vi "TimedCaseIndex.vi"(10 "CaseTimes":u32[](array[numeric]), 11 "ElapsedTime":u32) -> (3 "CaseNumber":u32)   [LabVIEW 2017]
panel:
  out "Numeric":i32
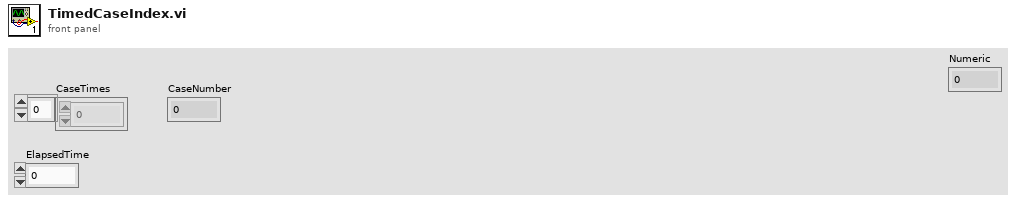
[diagram p1: front panel]
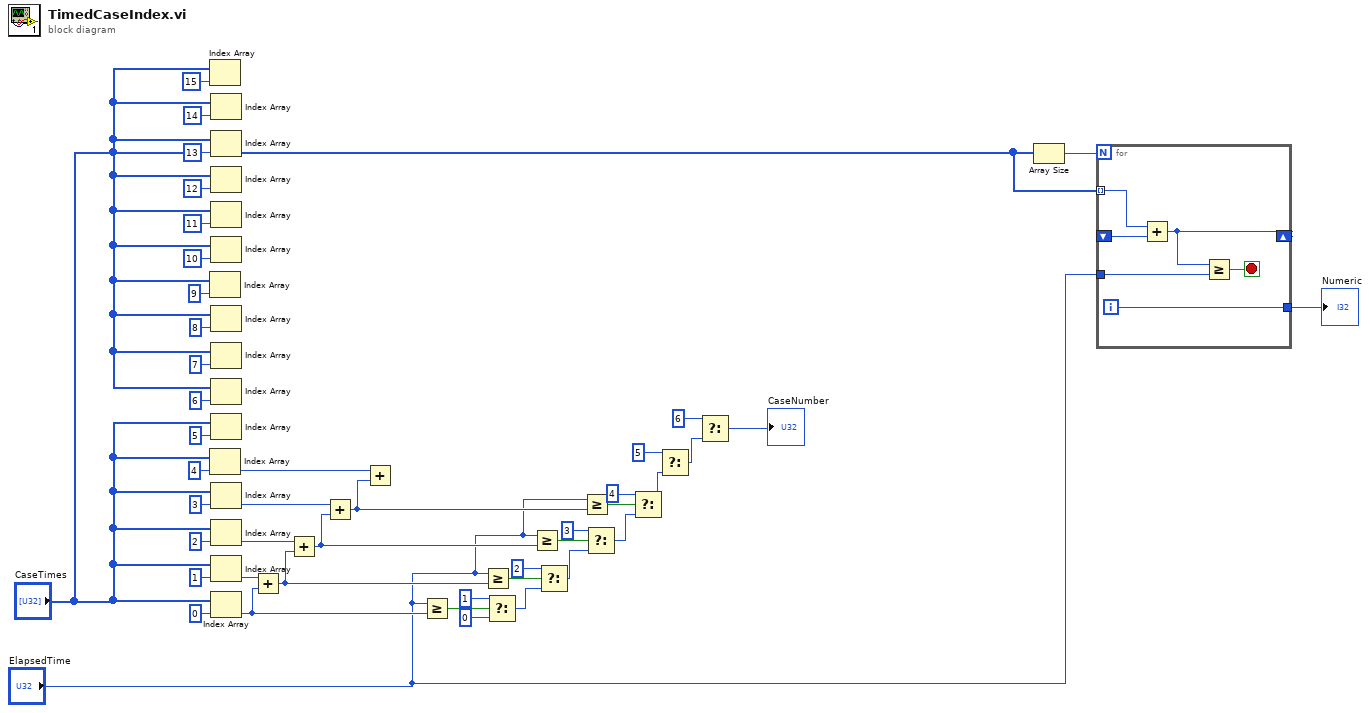
[diagram p0: block diagram]
diagram:
  n1 = Index Array(array="CaseTimes", index=15) -> ()  [unwired: 1 out]
  n2 = Index Array(array="CaseTimes", index=9) -> ()  [unwired: 1 out]
  n3 = Index Array(array="CaseTimes", index=4) -> (element=w6:u32)
  n4 = Index Array(array="CaseTimes", index=14) -> ()  [unwired: 1 out]
  n5 = Index Array(array="CaseTimes", index=13) -> ()  [unwired: 1 out]
  n6 = Index Array(array="CaseTimes", index=12) -> ()  [unwired: 1 out]
  n7 = Index Array(array="CaseTimes", index=11) -> ()  [unwired: 1 out]
  n8 = Index Array(array="CaseTimes", index=10) -> ()  [unwired: 1 out]
  n9 = Index Array(array="CaseTimes", index=8) -> ()  [unwired: 1 out]
  n10 = Index Array(array="CaseTimes", index=7) -> ()  [unwired: 1 out]
  n11 = Index Array(array="CaseTimes", index=6) -> ()  [unwired: 1 out]
  n12 = Index Array(array="CaseTimes", index=5) -> ()  [unwired: 1 out]
  n13 = Index Array(array="CaseTimes", index=3) -> (element=w10:u32)
  n14 = Index Array(array="CaseTimes", index=2) -> (element=w12:u32)
  n15 = Index Array(array="CaseTimes", index=1) -> (element=w15:u32)
  n16 = Index Array(array="CaseTimes", index=0) -> (element=w16:u32)
  n17 = Add(x=w15, y=w16) -> (x+y=w11:u32)
  n18 = Add(x=w12, y=w11) -> (x+y=w9:u32)
  n19 = Add(x=w10, y=w9) -> (x+y=w5:u32)
  n20 = Add(x=w6, y=w5) -> ()  [unwired: 1 out]
  n21 = Greater Or Equal?(x="ElapsedTime", y=w16) -> (x >= y?=w14:bool)
  n22 = Greater Or Equal?(x="ElapsedTime", y=w11) -> (x >= y?=w13:bool)
  n23 = Select(t=u32 1, s=w14, f=u32 0) -> (s? t:f=w41:u32)
  n24 = Greater Or Equal?(x="ElapsedTime", y=w9) -> (x >= y?=w8:bool)
  n25 = Select(t=u32 2, s=w13, f=w41) -> (s? t:f=w31:u32)
  n26 = Greater Or Equal?(x="ElapsedTime", y=w5) -> (x >= y?=w7:bool)
  n27 = Select(t=u32 3, s=w8, f=w31) -> (s? t:f=w32:u32)
  n28 = Select(t=u32 4, s=w7, f=w32) -> (s? t:f=w33:u32)
  n29 = Select(t=u32 5, f=w33) -> (s? t:f=w27:u32)  [unwired: 1 in]
  n30 = Select(t=u32 6, f=w27) -> (s? t:f=→"CaseNumber":u32)  [unwired: 1 in]
  n31 = Array Size(array="CaseTimes") -> (size(s)=w4:i32)
  n32 = for {
    N: w4 -> [_]
    shift-right: [w48] -> _
    shift-left: _ -> [w50]
    tunnel: "ElapsedTime" -> [w47]
    tunnel: "CaseTimes" -> [w51] mode=indexing
    tunnel: [w49] -> w1
    i -> [w49]
    stop <- w46 stop-if-true
    n33 = Add(x=w51, y=w50) -> (x+y=w48:u32)
    n34 = Greater Or Equal?(x=w48, y=w47) -> (x >= y?=w46:bool)
  }
  "Numeric" <- w1
